vi "LVClass_WavefrontCorrector Move Actuator to Absolute Position.vi"(0 "WavefrontCorrector in":refnum<class "WavefrontCorrector.lvclass">, 5 "Index of actuator":i32, 7 "Position":sgl, 11 "error in (no error)":errorcluster) -> (4 "WavefrontCorrector out":refnum<class "WavefrontCorrector.lvclass">, 15 "error out":errorcluster)   [LabVIEW 2020, in "WavefrontCorrector.lvclass"]
doc: "Move to requested absolute position, clip according to current preferences.\n\n<B>correctorIn</B> : WavefrontCorrector object.\n<B>correctorOut</B> : WavefrontCorrector object.\n<B>actuator_index</B> : Index of the actuator.\n<B>position</B> : Requested absolutes positions."
uses:
  WavefrontCorrector.lvclass
  WavefrontCorrector.lvclass/WavefrontCorrector.ctl
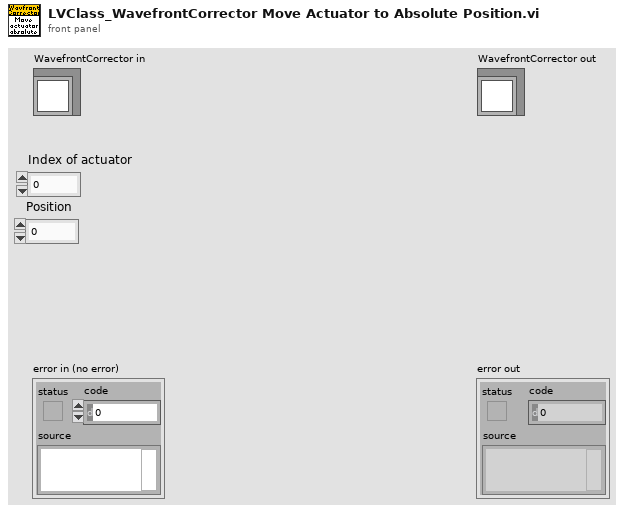
[diagram p1: front panel]
types:
  T1 = typedef "ClassID.ctl" = i64
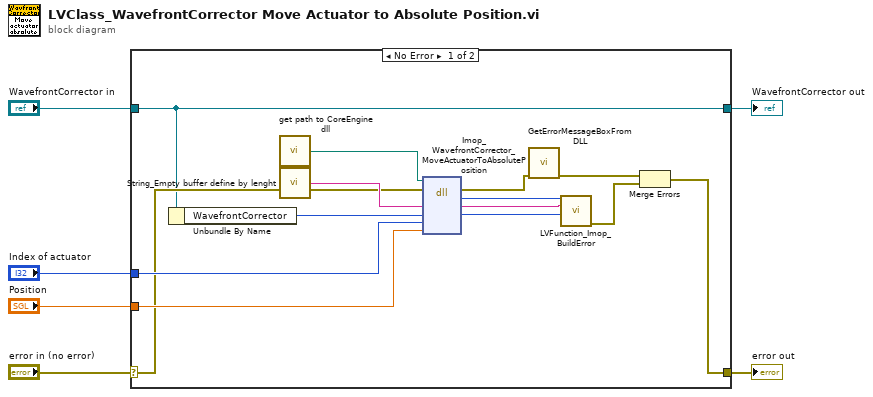
[diagram p0: block diagram]
diagram:
  n1 = case shown="No Error" "error in (no error)" {
    selector: "error in (no error)" -> [w10 w22]
    tunnel: [w11 w22] -> w5
    tunnel: [w9 w21] -> w3
    tunnel: "WavefrontCorrector in" -> [w9 w21]
    tunnel: "Index of actuator" -> [w13 _]
    tunnel: "Position" -> [w12 _]
    frame No Error {
      n2 = Unbundle By Name(w9) -> ("WavefrontCorrector"=w8:T1)
      n3 = call "get path to CoreEngine dll.vi"() -> ("path to wavekit library"=w14:path)  [unwired: 14 in, 1 out]
      n4 = call "String_Empty buffer define by lenght.vi"() -> ("Empty buffer"=w15:string)  [unwired: 1 in]
      n5 = dll-call lib="D:/FLE/0.Code/CoreEngine4_Suite/LV2011_interface/DLLs/c_interface_vc100.dll" fn="Imop_WavefrontCorrector_MoveActuatorToAbsolutePosition"(path in=w14, error in=w10, "Message"=w15, "WavefrontCorrector"=w8, "Index of actuator"=w13, "Position"=w12) -> (error out=w16:errorcluster, "return type"=w19:i32, "Message"=w20:string, "WavefrontCorrector"=w7:i64)  [unwired: 3 in, 1 out]
      n6 = call "GetErrorMessageBoxFromDLL.vi"("error IN"=w16) -> ("error OUT"=w17:errorcluster)  [unwired: 10 in]
      n7 = call "LVFunction_Imop_BuildError.vi"("code"=w19, "String to Prepend to source (\"\")"=w20, "Adresse"=w7) -> ("error out"=w18:errorcluster)  [unwired: 12 in]
      n8 = Merge Errors(w17, w18) -> (w11:errorcluster)
    }
    frame Error {
    }
  }
  "error out" <- w5
  "WavefrontCorrector out" <- w3
